vi "Modify pass.vi"(0 "vi path":path) -> ()   [LabVIEW 2015]
panel:
  out "appended array":bool[](array[boolean])
  out "User Name 2":string caption="User Name"
  in  "Exit Modify":bool
  in  "Replace":bool
  in  "New Password":string
  in  "New Name":string
  in  "New Group":u16(ring) items=["admin", "user"]
  in  "Delete":bool
  out "Contents":string[][](array[string])
  in  "Exit":bool
  in  "Modify":bool
  out "Password":string
  in  "User Name":string
  out "Group":u16(ring) items=["admin", "user"]
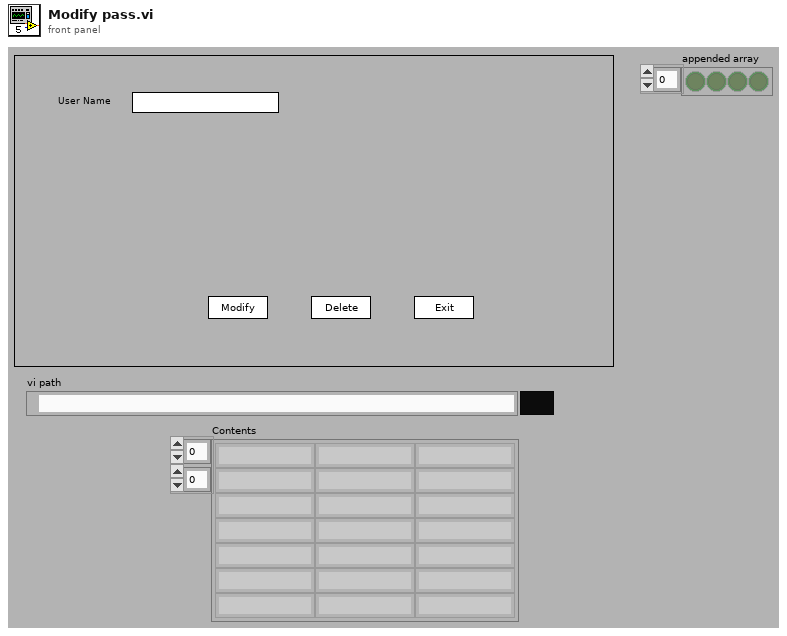
[diagram p1: front panel]
types:
  T1 = enum16{"open", "open or create", "create or replace", "create", "open (read only)"}
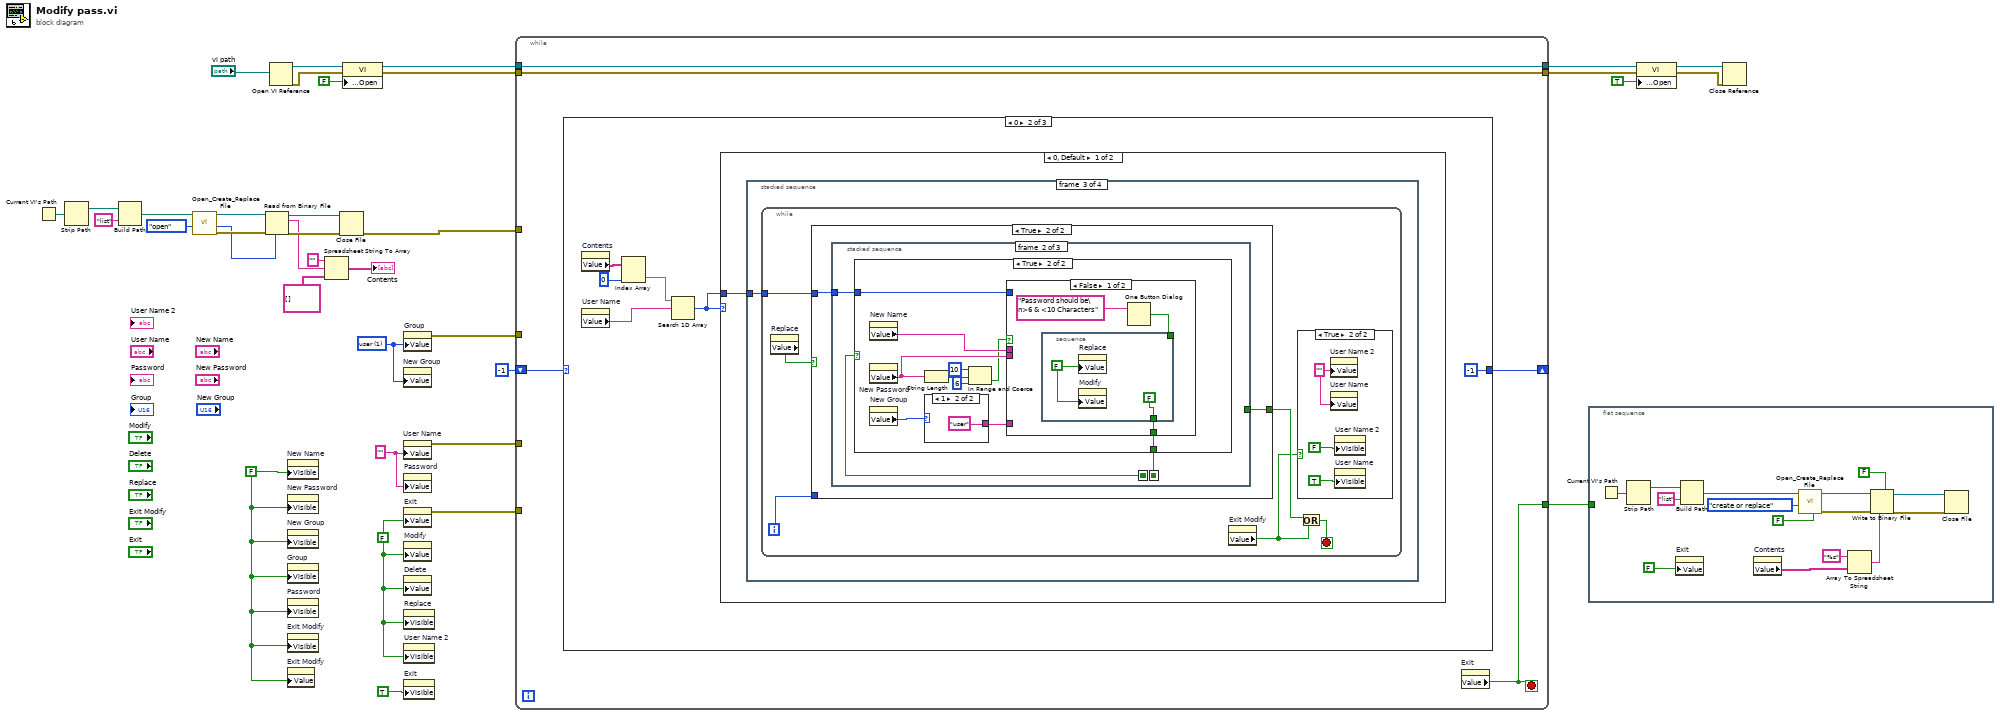
[diagram p0: block diagram]
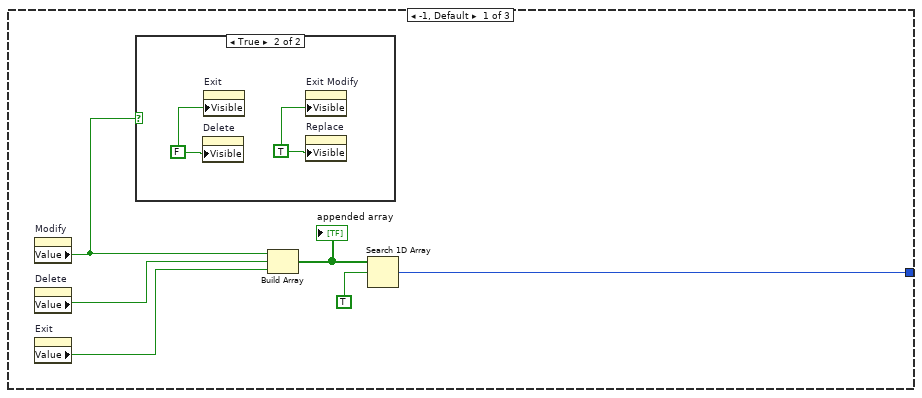
[diagram p2: hidden frame]
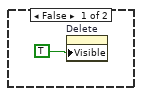
[diagram p3: hidden frame]
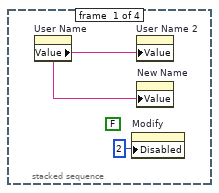
[diagram p4: hidden frame]
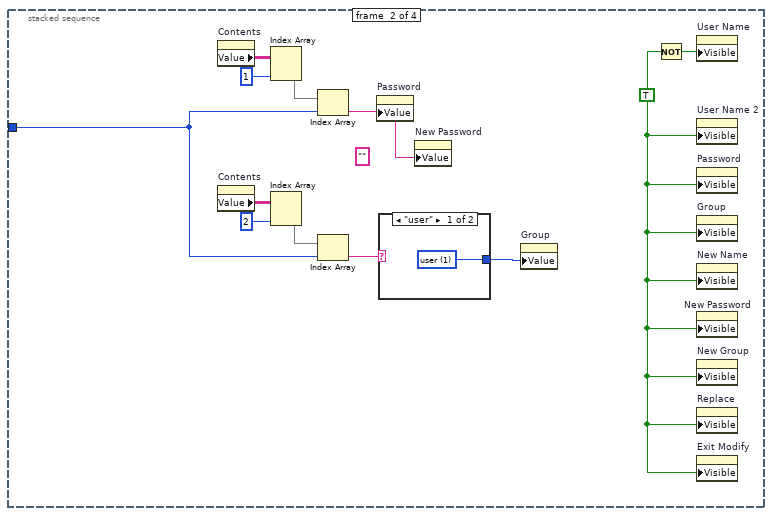
[diagram p5: hidden frame]
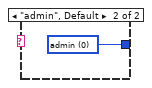
[diagram p6: hidden frame]
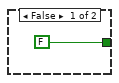
[diagram p8: hidden frame]
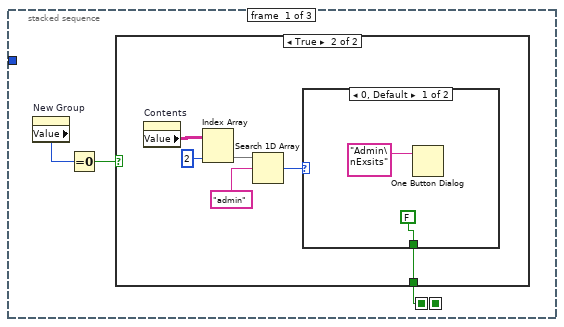
[diagram p9: hidden frame]
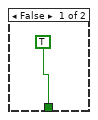
[diagram p10: hidden frame]
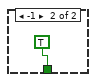
[diagram p11: hidden frame]
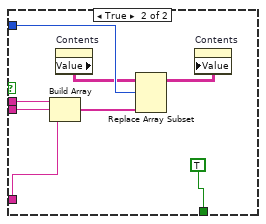
[diagram p13: hidden frame]
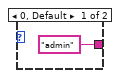
[diagram p14: hidden frame]
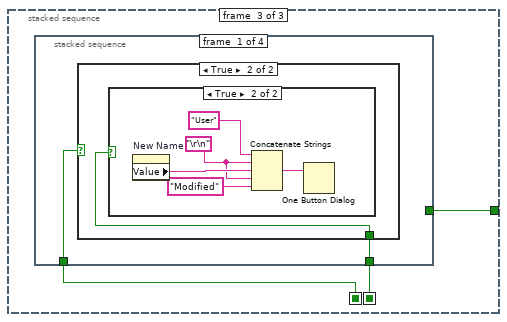
[diagram p15: hidden frame]
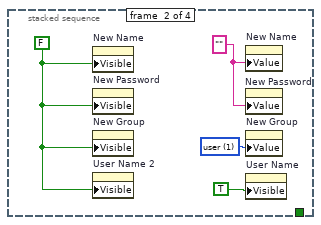
[diagram p18: hidden frame]
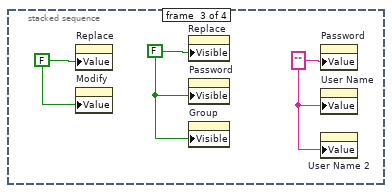
[diagram p19: hidden frame]
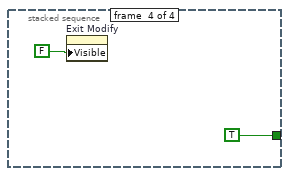
[diagram p20: hidden frame]
diagram:
  w5 = FALSE ("Visible")
  w20 = u16 1 items=["admin", "user"] ("Group")
  w6 = FALSE ("ADD")
  w25 = "" ("User Name")
  n1 = Current VI's Path() -> (path=w4:path)
  n2 = Strip Path(path=w4) -> (stripped path=w3:path)  [unwired: 1 out]
  n3 = Build Path(base path=w3, name or relative path="list") -> (appended path=w1:path)
  n4 = call <vilib>:"Open_Create_Replace File.vi"("function (open:0)"=T1."open", "file path"=w1) -> ("error out"=w36:errorcluster, "file size (bytes)"=w32:i32, "refnum"=w35:refnum<file>)  [unwired: 6 in, 1 out]
  n5 = Read from Binary File(8:w36, 10:w32, 11:w35) -> (0:w34:errorcluster, 2:w31:string, 3:w33:refnum<file>)  [unwired: 3 in, 1 out]
  n6 = Open VI Reference(vi path="vi path") -> (vi reference=w17:refnum<vi>, error out=w16:errorcluster)  [unwired: 5 in]
  n7 = property on="New Name" class="Str"("Visible"=w5) -> ()  [unwired: 2 in, 2 out]
  n8 = property on="New Password" class="Str"("Visible"=w5) -> ()  [unwired: 2 in, 2 out]
  n9 = property on="New Group" class="Ring (strict)"("Visible"=w5) -> ()  [unwired: 2 in, 2 out]
  n10 = property on="Group" class="Ring (strict)"("Visible"=w5) -> ()  [unwired: 2 in, 2 out]
  n11 = property on="Password" class="Str"("Visible"=w5) -> ()  [unwired: 2 in, 2 out]
  n12 = property on="Exit Modify" class="Bool (strict)"("Visible"=w5) -> ()  [unwired: 2 in, 2 out]
  n13 = property on="Exit Modify" class="Bool (strict)"("Value"=w5) -> ()  [unwired: 2 in, 2 out]
  n14 = Spreadsheet String To Array(format string="", spreadsheet string=w31, array type (2D Dbl)=string[][] []) -> (array=→"Contents":string[][])  [unwired: 1 in]
  n15 = Close File(refnum=w33, error in=w34) -> (error out=w26:errorcluster)  [unwired: 1 out]
  n16 = property class="VI"(reference=w17, error in=w16, "Front Panel Window:Open"=FALSE) -> (reference out=w14:refnum<vi>, error out=w13:errorcluster)
  n17 = property on="New Group" class="Ring (strict)"("Value"=w20) -> ()  [unwired: 2 in, 2 out]
  n18 = property on="User Name" class="Str"("Value"=w25) -> (error out=w24:errorcluster)  [unwired: 2 in, 1 out]
  n19 = property on="Group" class="Ring (strict)"("Value"=w20) -> (error out=w22:errorcluster)  [unwired: 2 in, 1 out]
  n20 = property on="Password" class="Str"("Value"=w25) -> ()  [unwired: 2 in, 2 out]
  n21 = property on="Exit" class="Bool (strict)"("Value"=w6) -> (error out=w7:errorcluster)  [unwired: 2 in, 1 out]
  n22 = property on="Modify" class="Bool (strict)"("Value"=w6) -> ()  [unwired: 2 in, 2 out]
  n23 = property on="Delete" class="Bool (strict)"("Value"=w6) -> ()  [unwired: 2 in, 2 out]
  n24 = property on="Replace" class="Bool (strict)"("Visible"=w6) -> ()  [unwired: 2 in, 2 out]
  n25 = property on="User Name 2" class="Str"("Visible"=w6) -> ()  [unwired: 2 in, 2 out]
  n26 = property on="Exit" class="Bool (strict)"("Visible"=TRUE) -> ()  [unwired: 2 in, 2 out]
  n27 = while {
    tunnel: w26 -> [_]
    tunnel: w24 -> [_]
    tunnel: [w41] -> w23
    tunnel: w22 -> [_]
    shift-right: [w40] -> _
    shift-left: -1 ("index of element") -> [w39]
    tunnel: w14 -> [w38]
    tunnel: w13 -> [w37]
    tunnel: [w38] -> w11
    tunnel: [w37] -> w10
    tunnel: w7 -> [_]
    stop <- w41 stop-if-true
    n28 = case shown="0" w39 {
      tunnel: [w43 -1 ("index of element") -1 ("index of element")] -> w40
      frame -1, Default {
        n29 = property on="Modify" class="Bool (strict)"() -> ("Value"=w42:bool)  [unwired: 2 in, 2 out]
        n30 = property on="Delete" class="Bool (strict)"() -> ("Value"=w47:bool)  [unwired: 2 in, 2 out]
        n31 = property on="Exit" class="Bool (strict)"() -> ("Value"=w46:bool)  [unwired: 2 in, 2 out]
        n32 = case shown="True" w42 {
          frame False {
            n33 = property on="Delete" class="Bool (strict)"("Visible"=TRUE) -> ()  [unwired: 2 in, 2 out]
          }
          frame True {
            w49 = FALSE ("Visible")
            w50 = TRUE ("Visible")
            n34 = property on="Delete" class="Bool (strict)"("Visible"=w49) -> ()  [unwired: 2 in, 2 out]
            n35 = property on="Exit" class="Bool (strict)"("Visible"=w49) -> ()  [unwired: 2 in, 2 out]
            n36 = property on="Exit Modify" class="Bool (strict)"("Visible"=w50) -> ()  [unwired: 2 in, 2 out]
            n37 = property on="Replace" class="Bool (strict)"("Visible"=w50) -> ()  [unwired: 2 in, 2 out]
          }
        }
        n38 = Build Array(w42, w47, w46) -> (w45:bool[])
        "appended array" <- w45
        n39 = Search 1D Array(1D array=w45, element=TRUE) -> (index of element=w43:i32)  [unwired: 1 in]
      }
      frame 0 {
        n40 = property on="Contents" class="Arr (strict)"() -> ("Value"=w55:string[][])  [unwired: 2 in, 2 out]
        n41 = property on="User Name" class="Str"() -> ("Value"=w53:string)  [unwired: 2 in, 2 out]
        n42 = Index Array(array=w55, index (col)=0 ("disabled index (col)")) -> (element=w51:string[])  [unwired: 1 in]
        n43 = Search 1D Array(1D array=w51, element=w53) -> (index of element=w52:i32)  [unwired: 1 in]
        n44 = case shown="0, Default" w52 {
          tunnel: w52 -> [w57 _]
          frame 0, Default {
            n45 = stacked-sequence {
              tunnel: w57 -> [_ w65 w74 _]
              frame #0 {
                (unwired) FALSE ("Visible")
                n46 = property on="User Name" class="Str"() -> ("Value"=w59:string)  [unwired: 2 in, 2 out]
                n47 = property on="Modify" class="Bool (strict)"("Disabled"=u8 2) -> ()  [unwired: 2 in, 2 out]
                n48 = property on="User Name 2" class="Str"("Value"=w59) -> ()  [unwired: 2 in, 2 out]
                n49 = property on="New Name" class="Str"("Value"=w59) -> ()  [unwired: 2 in, 2 out]
              }
              frame #1 {
                (unwired) "" ("New Password")
                w61 = TRUE ("Visible")
                n50 = property on="Contents" class="Arr (strict)"() -> ("Value"=w70:string[][])  [unwired: 2 in, 2 out]
                n51 = property on="Contents" class="Arr (strict)"() -> ("Value"=w67:string[][])  [unwired: 2 in, 2 out]
                n52 = Index Array(array=w70, index (col)=1 ("disabled index (col)")) -> (element=w69:string[])  [unwired: 1 in]
                n53 = Index Array(array=w67, index (col)=2 ("disabled index (col)")) -> (element=w68:string[])  [unwired: 1 in]
                n54 = Index Array(array=w69, index=w65) -> (element=w60:string)
                n55 = Index Array(array=w68, index=w65) -> (element=w64:string)
                n56 = property on="Password" class="Str"("Value"=w60) -> ()  [unwired: 2 in, 2 out]
                n57 = case shown="\"user\"" w64 {
                  tunnel: [w72 w73] -> w63
                  frame "user" {
                    w72 = u16 1 items=["admin", "user"] ("Group")
                  }
                  frame "admin", Default {
                    w73 = u16 0 items=["admin", "user"] ("Group")
                  }
                }
                n58 = property on="New Password" class="Str"("Value"=w60) -> ()  [unwired: 2 in, 2 out]
                n59 = property on="Group" class="Ring (strict)"("Value"=w63) -> ()  [unwired: 2 in, 2 out]
                n60 = Not(x=w61) -> (.not. x?=w62:bool)
                n61 = property on="User Name" class="Str"("Visible"=w62) -> ()  [unwired: 2 in, 2 out]
                n62 = property on="User Name 2" class="Str"("Visible"=w61) -> ()  [unwired: 2 in, 2 out]
                n63 = property on="Password" class="Str"("Visible"=w61) -> ()  [unwired: 2 in, 2 out]
                n64 = property on="Group" class="Ring (strict)"("Visible"=w61) -> ()  [unwired: 2 in, 2 out]
                n65 = property on="New Name" class="Str"("Visible"=w61) -> ()  [unwired: 2 in, 2 out]
                n66 = property on="New Password" class="Str"("Visible"=w61) -> ()  [unwired: 2 in, 2 out]
                n67 = property on="New Group" class="Ring (strict)"("Visible"=w61) -> ()  [unwired: 2 in, 2 out]
                n68 = property on="Replace" class="Bool (strict)"("Visible"=w61) -> ()  [unwired: 2 in, 2 out]
                n69 = property on="Exit Modify" class="Bool (strict)"("Visible"=w61) -> ()  [unwired: 2 in, 2 out]
              }
              frame #2 {
                n70 = while {
                  tunnel: w74 -> [w80]
                  i -> [w75]
                  stop <- w78 stop-if-true
                  n71 = property on="Replace" class="Bool (strict)"() -> ("Value"=w79:bool)  [unwired: 2 in, 2 out]
                  n72 = case shown="True" w79 {
                    tunnel: w80 -> [_ w86]
                    tunnel: [FALSE w85] -> w77
                    tunnel: w75 -> [_ _]
                    frame False {
                    }
                    frame True {
                      n73 = stacked-sequence {
                        seq-local: [w87 _ _] -> [_ w101 w129]
                        seq-local: [_ w100 _] -> [_ _ w128]
                        tunnel: w86 -> [_ w102 _]
                        tunnel: [_ _ w130] -> w85
                        frame #0 {
                          n74 = property on="New Group" class="Ring (strict)"() -> ("Value"=w89:u16)  [unwired: 2 in, 2 out]
                          n75 = Equal To 0?(x=w89) -> (x = 0?=w88:bool)
                          n76 = case shown="True" w88 {
                            tunnel: [TRUE w92] -> w87
                            frame False {
                            }
                            frame True {
                              n77 = property on="Contents" class="Arr (strict)"() -> ("Value"=w96:string[][])  [unwired: 2 in, 2 out]
                              n78 = Index Array(array=w96, index (col)=2 ("index (row)")) -> (element=w95:string[])  [unwired: 1 in]
                              n79 = Search 1D Array(1D array=w95, element="admin") -> (index of element=w93:i32)  [unwired: 1 in]
                              n80 = case shown="0, Default" w93 {
                                tunnel: [FALSE TRUE] -> w92
                                frame 0, Default {
                                n81 = One Button Dialog(message="Admin\nExsits") -> ()  [unwired: 1 in, 1 out]
                                }
                                frame -1 {
                                }
                              }
                            }
                          }
                        }
                        frame #1 {
                          n82 = case shown="True" w101 {
                            tunnel: w102 -> [_ w112]
                            tunnel: [_ w111] -> w100
                            frame False {
                            }
                            frame True {
                              n83 = property on="New Name" class="Str"() -> ("Value"=w109:string)  [unwired: 2 in, 2 out]
                              n84 = property on="New Password" class="Str"() -> ("Value"=w107:string)  [unwired: 2 in, 2 out]
                              n85 = property on="New Group" class="Ring (strict)"() -> ("Value"=w110:u16)  [unwired: 2 in, 2 out]
                              n86 = String Length(string=w107) -> (length=w106:i32)
                              n87 = case shown="1" w110 {
                                tunnel: ["admin" "user"] -> w108
                                frame 0, Default {
                                }
                                frame 1 {
                                }
                              }
                              n88 = In Range and Coerce(upper limit=10, x=w106, lower limit=6) -> (In Range?=w103:bool)  [unwired: 1 out]
                              n89 = case shown="False" w103 {
                                tunnel: w109 -> [_ w125]
                                tunnel: w112 -> [_ w124]
                                tunnel: w108 -> [_ w120]
                                tunnel: w107 -> [_ w119]
                                tunnel: [w114 TRUE ("Visible")] -> w111
                                frame False {
                                n90 = One Button Dialog(message="Password should be\n>6 & <10 Characters") -> (true=w113:bool)  [unwired: 1 in]
                                n91 = stacked-sequence {
                                tunnel: [FALSE ("Visible")] -> w114
                                tunnel: w113 -> [_]
                                frame #0 {
                                w117 = FALSE ("Visible")
                                n92 = property on="Replace" class="Bool (strict)"("Value"=w117) -> ()  [unwired: 2 in, 2 out]
                                n93 = property on="Modify" class="Bool (strict)"("Value"=w117) -> ()  [unwired: 2 in, 2 out]
                                }
                                }
                                }
                                frame True {
                                n94 = Build Array(w125, w119, w120) -> (w123:string[])
                                n95 = property on="Contents" class="Arr (strict)"() -> ("Value"=w122:string[][])  [unwired: 2 in, 2 out]
                                n96 = Replace Array Subset(array=w122, new element=w123, index (row)=w124) -> (w121:string[][])  [unwired: 1 in]
                                n97 = property on="Contents" class="Arr (strict)"("Value"=w121) -> ()  [unwired: 2 in, 2 out]
                                }
                              }
                            }
                          }
                        }
                        frame #2 {
                          n98 = stacked-sequence {
                            tunnel: [_ _ _ TRUE ("Visible")] -> w130
                            tunnel: w129 -> [w132 _ _ _]
                            tunnel: w128 -> [w131 _ _ _]
                            frame #0 {
                              n99 = case shown="True" w132 {
                                tunnel: w131 -> [_ w133]
                                frame False {
                                }
                                frame True {
                                n100 = case shown="True" w133 {
                                frame False {
                                }
                                frame True {
                                w136 = "\r\n"
                                n101 = property on="New Name" class="Str"() -> ("Value"=w137:string)  [unwired: 2 in, 2 out]
                                n102 = Concatenate Strings("User" ("string"), w136, w137, w136, "Modified" ("string")) -> (w134:string)
                                n103 = One Button Dialog(message=w134) -> ()  [unwired: 1 in, 1 out]
                                }
                                }
                                }
                              }
                            }
                            frame #1 {
                              w141 = u16 1 items=["admin", "user"] ("New Group")
                              w142 = ""
                              w140 = FALSE
                              n104 = property on="New Name" class="Str"("Visible"=w140) -> ()  [unwired: 2 in, 2 out]
                              n105 = property on="New Password" class="Str"("Visible"=w140) -> ()  [unwired: 2 in, 2 out]
                              n106 = property on="New Group" class="Ring (strict)"("Visible"=w140) -> ()  [unwired: 2 in, 2 out]
                              n107 = property on="User Name 2" class="Str"("Visible"=w140) -> ()  [unwired: 2 in, 2 out]
                              n108 = property on="New Name" class="Str"("Value"=w142) -> ()  [unwired: 2 in, 2 out]
                              n109 = property on="New Password" class="Str"("Value"=w142) -> ()  [unwired: 2 in, 2 out]
                              n110 = property on="New Group" class="Ring (strict)"("Value"=w141) -> ()  [unwired: 2 in, 2 out]
                              n111 = property on="User Name" class="Str"("Visible"=TRUE) -> ()  [unwired: 2 in, 2 out]
                            }
                            frame #2 {
                              w145 = FALSE ("Visible")
                              w143 = "" ("Password")
                              w144 = FALSE ("Replace")
                              n112 = property on="Replace" class="Bool (strict)"("Value"=w144) -> ()  [unwired: 2 in, 2 out]
                              n113 = property on="Modify" class="Bool (strict)"("Value"=w144) -> ()  [unwired: 2 in, 2 out]
                              n114 = property on="Replace" class="Bool (strict)"("Visible"=w145) -> ()  [unwired: 2 in, 2 out]
                              n115 = property on="Password" class="Str"("Visible"=w145) -> ()  [unwired: 2 in, 2 out]
                              n116 = property on="Group" class="Ring (strict)"("Visible"=w145) -> ()  [unwired: 2 in, 2 out]
                              n117 = property on="Password" class="Str"("Value"=w143) -> ()  [unwired: 2 in, 2 out]
                              n118 = property on="User Name" class="Str"("Value"=w143) -> ()  [unwired: 2 in, 2 out]
                              n119 = property on="User Name 2" class="Str"("Value"=w143) -> ()  [unwired: 2 in, 2 out]
                            }
                            frame #3 {
                              n120 = property on="Exit Modify" class="Bool (strict)"("Visible"=FALSE) -> ()  [unwired: 2 in, 2 out]
                            }
                          }
                        }
                      }
                    }
                  }
                  n121 = property on="Exit Modify" class="Bool (strict)"() -> ("Value"=w76:bool)  [unwired: 2 in, 2 out]
                  n122 = case shown="True" w76 {
                    frame False {
                    }
                    frame True {
                      w81 = "" ("User Name 2")
                      n123 = property on="User Name 2" class="Str"("Value"=w81) -> ()  [unwired: 2 in, 2 out]
                      n124 = property on="User Name" class="Str"("Value"=w81) -> ()  [unwired: 2 in, 2 out]
                      n125 = property on="User Name 2" class="Str"("Visible"=FALSE) -> ()  [unwired: 2 in, 2 out]
                      n126 = property on="User Name" class="Str"("Visible"=TRUE) -> ()  [unwired: 2 in, 2 out]
                    }
                  }
                  n127 = Or(x=w77, y=w76) -> (x .or. y?=w78:bool)
                }
              }
              frame #3 {
                w151 = FALSE ("Modify")
                w153 = u16 1 items=["admin", "user"] ("New Group")
                w154 = ""
                w150 = FALSE
                w152 = FALSE ("Visible")
                w149 = TRUE ("Visible")
                n128 = property on="Modify" class="Bool (strict)"("Disabled"=u8 0) -> ()  [unwired: 2 in, 2 out]
                n129 = property on="Delete" class="Bool (strict)"("Visible"=w149) -> ()  [unwired: 2 in, 2 out]
                n130 = property on="Exit" class="Bool (strict)"("Visible"=w149) -> ()  [unwired: 2 in, 2 out]
                n131 = property on="New Name" class="Str"("Value"=w154) -> ()  [unwired: 2 in, 2 out]
                n132 = property on="New Password" class="Str"("Value"=w154) -> ()  [unwired: 2 in, 2 out]
                n133 = property on="New Group" class="Ring (strict)"("Value"=w153) -> ()  [unwired: 2 in, 2 out]
                n134 = property on="Modify" class="Bool (strict)"("Value"=w151) -> ()  [unwired: 2 in, 2 out]
                n135 = property on="Exit Modify" class="Bool (strict)"("Value"=w151) -> ()  [unwired: 2 in, 2 out]
                n136 = property on="Replace" class="Bool (strict)"("Visible"=w152) -> ()  [unwired: 2 in, 2 out]
                n137 = property on="Exit Modify" class="Bool (strict)"("Visible"=w152) -> ()  [unwired: 2 in, 2 out]
                n138 = property on="New Name" class="Str"("Visible"=w150) -> ()  [unwired: 2 in, 2 out]
                n139 = property on="Password" class="Str"("Visible"=w150) -> ()  [unwired: 2 in, 2 out]
                n140 = property on="New Password" class="Str"("Visible"=w150) -> ()  [unwired: 2 in, 2 out]
                n141 = property on="Group" class="Ring (strict)"("Visible"=w150) -> ()  [unwired: 2 in, 2 out]
                n142 = property on="New Group" class="Ring (strict)"("Visible"=w150) -> ()  [unwired: 2 in, 2 out]
              }
            }
          }
          frame -1 {
            n143 = stacked-sequence {
              frame #0 {
                n144 = One Button Dialog(message="User Name \n Not Found") -> ()  [unwired: 1 in, 1 out]
              }
              frame #1 {
                w157 = FALSE ("ADD")
                n145 = property on="Exit" class="Bool (strict)"("Visible"=TRUE) -> ()  [unwired: 2 in, 2 out]
                n146 = property on="Modify" class="Bool (strict)"("Value"=w157) -> ()  [unwired: 2 in, 2 out]
                n147 = property on="Exit Modify" class="Bool (strict)"("Visible"=w157) -> ()  [unwired: 2 in, 2 out]
                n148 = property on="Password" class="Str"("Visible"=w157) -> ()  [unwired: 2 in, 2 out]
                n149 = property on="Group" class="Ring (strict)"("Visible"=w157) -> ()  [unwired: 2 in, 2 out]
                n150 = property on="Replace" class="Bool (strict)"("Visible"=w157) -> ()  [unwired: 2 in, 2 out]
                n151 = property on="New Name" class="Str"("Visible"=w157) -> ()  [unwired: 2 in, 2 out]
                n152 = property on="New Password" class="Str"("Visible"=w157) -> ()  [unwired: 2 in, 2 out]
                n153 = property on="New Group" class="Ring (strict)"("Visible"=w157) -> ()  [unwired: 2 in, 2 out]
              }
              frame #2 {
                w158 = "" ("User Name")
                n154 = property on="User Name" class="Str"("Value"=w158) -> ()  [unwired: 2 in, 2 out]
                n155 = property on="Password" class="Str"("Value"=w158) -> ()  [unwired: 2 in, 2 out]
              }
            }
          }
        }
      }
      frame 1 {
        n156 = property on="Contents" class="Arr (strict)"() -> ("Value"=w164:string[][])  [unwired: 2 in, 2 out]
        n157 = property on="User Name" class="Str"() -> ("Value"=w161:string)  [unwired: 2 in, 2 out]
        n158 = Index Array(array=w164, index (col)=0 ("disabled index (col)")) -> (element=w162:string[])  [unwired: 1 in]
        n159 = Search 1D Array(1D array=w162, element=w161) -> (index of element=w160:i32)  [unwired: 1 in]
        n160 = case shown="0, Default" w160 {
          tunnel: w160 -> [w165 _]
          frame 0, Default {
            n161 = stacked-sequence {
              seq-local: [w166 _ _] -> [_ w174 _]
              tunnel: w165 -> [_ w173 _]
              frame #0 {
                n162 = property on="User Name" class="Str"() -> ("Value"=w172:string)  [unwired: 2 in, 2 out]
                n163 = Concatenate Strings(w172, "\r\n", "Confirm Delete" ("string")) -> (w169:string)
                n164 = Two Button Dialog(message=w169, 1:"Cancel" ("T button name (\"OK\")"), 2:"Delete" ("T button name (\"OK\")")) -> (T button?=w166:bool)
              }
              frame #1 {
                n165 = case shown="True" w174 {
                  tunnel: w173 -> [_ w179]
                  frame False {
                    n166 = property on="User Name" class="Str"("Value"="" ("User Name")) -> ()  [unwired: 2 in, 2 out]
                  }
                  frame True {
                    n167 = property on="Contents" class="Arr (strict)"() -> ("Value"=w180:string[][])  [unwired: 2 in, 2 out]
                    n168 = Delete From Array(array=w180, index (row)=w179) -> (array with subset deleted=w178:string[][])  [unwired: 2 in, 1 out]
                    n169 = property on="Contents" class="Arr (strict)"("Value"=w178) -> (error out=w176:errorcluster)  [unwired: 2 in, 1 out]
                    n170 = property on="User Name" class="Str"(error in=w176, "Value"="" ("User Name")) -> ()  [unwired: 1 in, 2 out]
                  }
                }
              }
              frame #2 {
                n171 = property on="Delete" class="Bool (strict)"("Value"=FALSE ("Delete")) -> ()  [unwired: 2 in, 2 out]
              }
            }
          }
          frame -1 {
            n172 = stacked-sequence {
              frame #0 {
                n173 = property on="User Name" class="Str"() -> ("Value"=w184:string)  [unwired: 2 in, 2 out]
                n174 = Concatenate Strings(w184, "\r\n", "Not Found" ("string")) -> (w185:string)
                n175 = One Button Dialog(message=w185) -> ()  [unwired: 1 in, 1 out]
              }
              frame #1 {
                n176 = property on="Delete" class="Bool (strict)"("Value"=FALSE ("Delete")) -> ()  [unwired: 2 in, 2 out]
              }
            }
          }
        }
      }
    }
    n177 = property on="Exit" class="Bool (strict)"() -> ("Value"=w41:bool)  [unwired: 2 in, 2 out]
  }
  n178 = flat-sequence {
    tunnel: w23 -> [_]
    frame #0 {
      n179 = Current VI's Path() -> (path=w191:path)
      n180 = Strip Path(path=w191) -> (stripped path=w190:path)  [unwired: 1 out]
      n181 = property on="Exit" class="Bool (strict)"("Value"=FALSE ("ADD")) -> ()  [unwired: 2 in, 2 out]
      n182 = Build Path(base path=w190, name or relative path="list") -> (appended path=w188:path)
      n183 = property on="Contents" class="Arr (strict)"() -> ("Value"=w196:string[][])  [unwired: 2 in, 2 out]
      n184 = call <vilib>:"Open_Create_Replace File.vi"("advisory dialog? (display:T)"=FALSE, "function (open:0)"=T1."create or replace", "file path"=w188) -> ("error out"=w197:errorcluster, "refnum"=w198:refnum<file>)  [unwired: 5 in, 2 out]
      n185 = Array To Spreadsheet String(array=w196, 3:"%s" ("format string")) -> (spreadsheet string=w195:string)  [unwired: 1 in]
      n186 = Write to Binary File(file (use dialog)=w198, data=w195, error in=w197, 5:FALSE ("prepend array or string size? (T)")) -> (refnum out=w200:refnum<file>, error out=w199:errorcluster)  [unwired: 2 in, 1 out]
      n187 = Close File(refnum=w200, error in=w199) -> ()  [unwired: 2 out]
    }
  }
  n188 = property class="VI"(reference=w11, error in=w10, "Front Panel Window:Open"=TRUE) -> (reference out=w9:refnum<vi>, error out=w8:errorcluster)
  n189 = Close Reference(reference=w9, error in (no error)=w8) -> ()  [unwired: 1 out]
